vi "XY Graph Special Event Handler Wrapper.vi"(8 "Error In":errorcluster, 11 "XY Graph Event":T1) -> (0 "Error Out":errorcluster, 3 "Message":string)   [LabVIEW 2019, in "XY Graph Add-Ons.lvlib"]
uses:
  XY Graph Add-Ons.lvlib
  XY Graph Event.ctl
  <vilib>/Utility/miscctls.llb/LVPoint32TypeDef.ctl
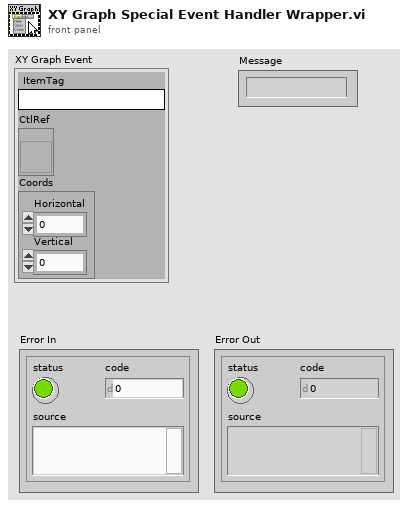
[diagram p1: front panel]
types:
  T1 = typedef "XY Graph Event.ctl" = cluster{"ItemTag":string, "CtlRef":refnum<vi>, "Coords":T2}
  T2 = typedef "LVPoint32TypeDef.ctl" = cluster{"Horizontal":i32, "Vertical":i32}
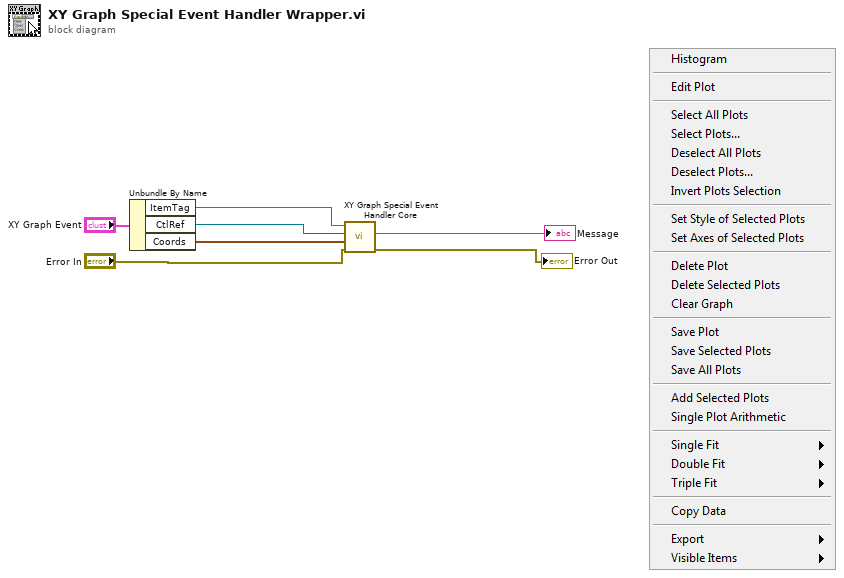
[diagram p0: block diagram]
diagram:
  n1 = Unbundle By Name("XY Graph Event") -> ("ItemTag"=w2:string, "CtlRef"=w3:refnum<vi>, "Coords"=w6:T2)
  n2 = call "XY Graph Special Event Handler Core.vi"("error in (no error)"="Error In", "Coords"=w6, "XYGraph in"=w3, "ItemTag"=w2) -> ("error out"=→"Error Out":errorcluster, "Message"=→"Message":string)  [unwired: 6 in]
